vi "Calculate_Global_Cost_F()-3.vi"(6 "[IN] Max angle":dbl, 7 "[IN] Subtracks in Row":T1(array[cluster]), 8 "error IN":errorcluster, 9 "[IN] Areas particles\nPrimary Detected":dbl[][](array[numeric]), 10 "[IN] Primary \n(X,Y) Detected":dbl[][](array[numeric]), 11 "[IN] Cost function":i8[](array[numeric])) -> (0 "error OUT":errorcluster, 3 "[OUT] Cost function":i8[](array[numeric]))   [LabVIEW 2013]
uses:
  <vilib>/Analysis/NI_AALBase.lvlib
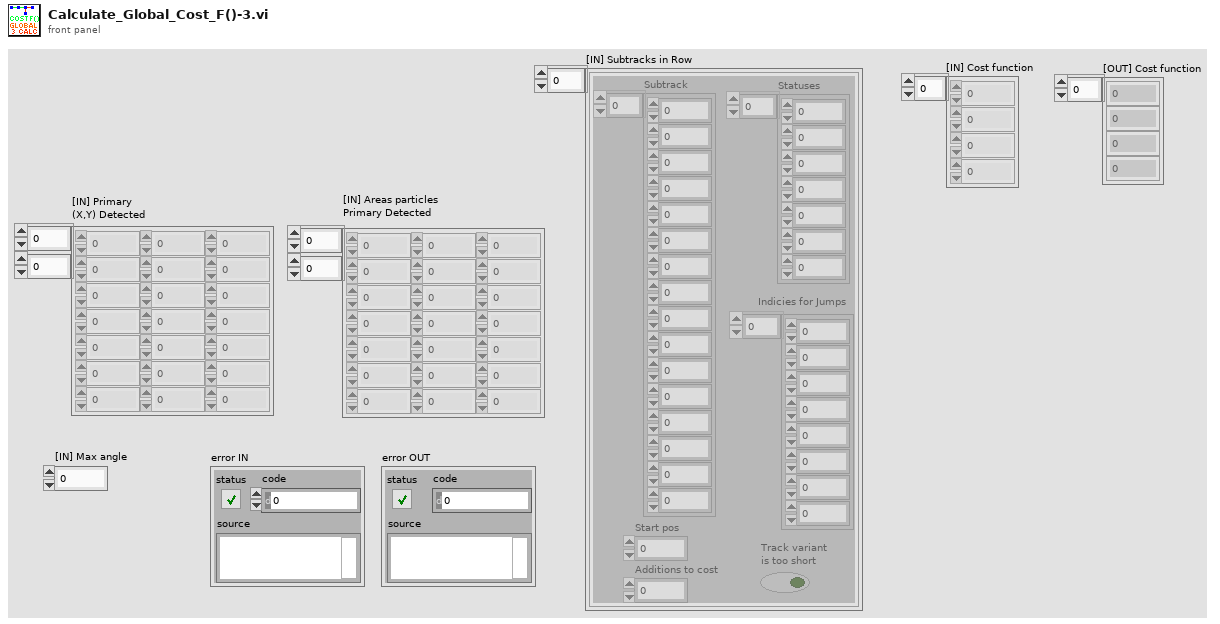
[diagram p1: front panel]
types:
  T1 = cluster{"Subtrack":dbl[], "Statuses":i16[], "Start pos":i32, "Additions to cost":i8, "Track variant \nis too short":bool, "Indicies for Jumps":i32[]}[]
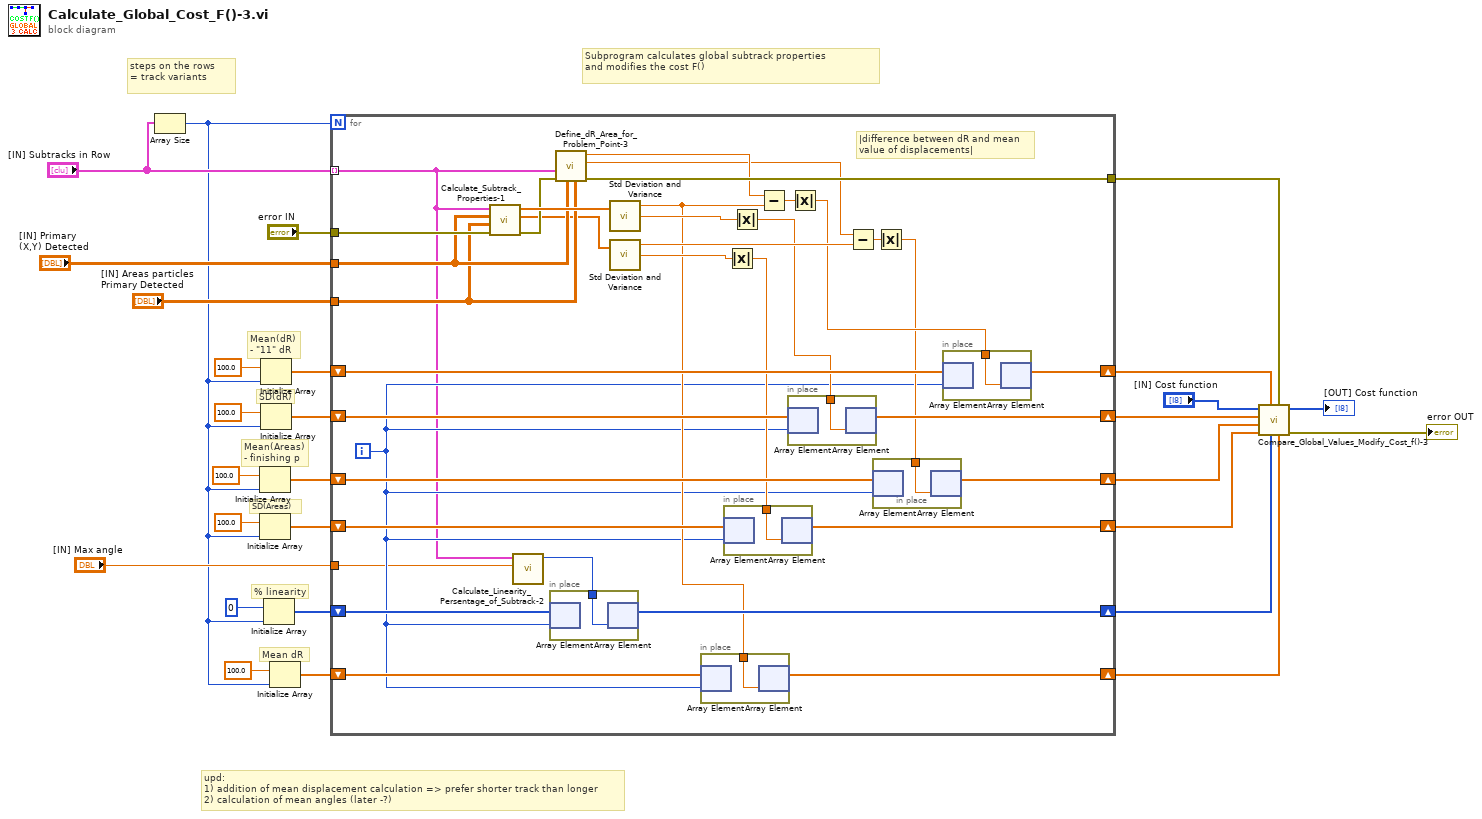
[diagram p0: block diagram]
diagram:
  # "upd: \n1) addition of mean displacement calculation => prefer shorter track than longer \n2) calculation of mean angles (later -?)"
  # "Mean dR"
  # "Subprogram calculates global subtrack properties\nand modifies the cost F()"
  # "Mean(Areas)\n- finishing p"
  # "SD(Areas)"
  # "% linearity"
  # "Mean(dR)\n- \"11\" dR"
  # "SD(dR)"
  # "steps on the rows\n= track variants"
  n1 = Array Size(array="[IN] Subtracks in Row") -> (size(s)=w3:i32)
  n2 = Initialize Array(100.0, w3) -> (w18:dbl[])
  n3 = Initialize Array(100.0, w3) -> (w17:dbl[])
  n4 = Initialize Array(100.0, w3) -> (w26:dbl[])
  n5 = Initialize Array(100.0, w3) -> (w25:dbl[])
  n6 = Initialize Array(u8 0, w3) -> (w15:u8[])
  n7 = Initialize Array(100.0, w3) -> (w2:dbl[])
  n8 = for {
    N: w3 -> [_]
    shift-right: [w48] -> w12
    shift-left: w26 -> [w49]
    shift-right: [w45] -> w5
    shift-left: w25 -> [w47]
    tunnel: "error IN" -> [w63]
    tunnel: "[IN] Primary \n(X,Y) Detected" -> [w53]
    tunnel: "[IN] Areas particles\nPrimary Detected" -> [w52]
    shift-right: [w42] -> w6
    shift-left: w18 -> [w44]
    shift-right: [w39] -> w7
    shift-left: w17 -> [w41]
    tunnel: "[IN] Max angle" -> [w30]
    shift-right: [w37] -> w8
    shift-left: w15 -> [w38]
    tunnel: [w55] -> w11
    tunnel: "[IN] Subtracks in Row" -> [w31] mode=indexing
    shift-right: [w33] -> w1
    shift-left: w2 -> [w35]
    i -> [w32]
    # "|difference between dR and mean\nvalue of displacements|"
    n9 = call "Calculate_Subtrack_Properties-1.vi"("error IN"=w63, "[IN] Areas particles\nPrimary Detected"=w52, "[IN] Primary \n(X,Y) Detected"=w53, "[IN] Subtrack"=w31) -> ("error OUT"=w56:errorcluster, "[OUT] Areas"=w36:dbl[], "[OUT] dR (displ)"=w62:dbl[])  [unwired: 2 in, 1 out]
    n10 = call "Calculate_Linearity_Persentage_of_Subtrack-2.vi"("[IN] Max angle"=w30, "[IN] Subtrack"=w31) -> ("[OUT] Track Linearity in %"=w29:u8)  [unwired: 5 in]
    n11 = in-place {
      in-place-border: w29 -> [w65]
      n12 = in-place-array #1(w38, w32) -> ()  [unwired: 1 out]
      n13 = in-place-array #1(w65) -> (w37:u8[])  [unwired: 1 out]
    }
    n14 = call "Define_dR_Area_for_Problem_Point-3.vi"("[IN] Areas particles\nPrimary Detected"=w52, "[IN] Primary \n(X,Y) Detected"=w53, "error IN"=w56, "[IN] Subtrack"=w31) -> ("error OUT"=w55:errorcluster, "[OUT] Area Problem Point\n101 - Starting Point\n11 - Ending Point"=w51:dbl, "[OUT] dR for Problem Point"=w54:dbl)  [unwired: 5 in]
    n15 = call <vilib>:"Std Deviation and Variance.vi"("X"=w62) -> ("mean"=w34:dbl, "standard deviation"=w61:dbl)  [unwired: 1 in, 1 out]
    n16 = call <vilib>:"Std Deviation and Variance.vi"("X"=w36) -> ("mean"=w58:dbl, "standard deviation"=w60:dbl)  [unwired: 1 in, 1 out]
    n17 = in-place {
      in-place-border: w34 -> [w64]
      n18 = in-place-array #2(w35, w32) -> ()  [unwired: 1 out]
      n19 = in-place-array #2(w64) -> (w33:dbl[])  [unwired: 1 out]
    }
    n20 = Absolute Value(x=w60) -> (abs(x)=w40:dbl)
    n21 = in-place {
      in-place-border: w40 -> [w66]
      n22 = in-place-array #3(w41, w32) -> ()  [unwired: 1 out]
      n23 = in-place-array #3(w66) -> (w39:dbl[])  [unwired: 1 out]
    }
    n24 = Absolute Value(x=w61) -> (abs(x)=w46:dbl)
    n25 = Subtract(x=w54, y=w34) -> (x-y=w59:dbl)
    n26 = in-place {
      in-place-border: w46 -> [w68]
      n27 = in-place-array #4(w47, w32) -> ()  [unwired: 1 out]
      n28 = in-place-array #4(w68) -> (w45:dbl[])  [unwired: 1 out]
    }
    n29 = Absolute Value(x=w59) -> (abs(x)=w50:dbl)
    n30 = Subtract(x=w51, y=w58) -> (x-y=w57:dbl)
    n31 = Absolute Value(x=w57) -> (abs(x)=w43:dbl)
    n32 = in-place {
      in-place-border: w43 -> [w67]
      n33 = in-place-array #5(w44, w32) -> ()  [unwired: 1 out]
      n34 = in-place-array #5(w67) -> (w42:dbl[])  [unwired: 1 out]
    }
    n35 = in-place {
      in-place-border: w50 -> [w69]
      n36 = in-place-array #6(w49, w32) -> ()  [unwired: 1 out]
      n37 = in-place-array #6(w69) -> (w48:dbl[])  [unwired: 1 out]
    }
  }
  n38 = call "Compare_Global_Values_Modify_Cost_f()-3.vi"("[IN] Mean dR"=w1, "error IN"=w11, "[IN] Linearity"=w8, "[IN] Array of Mean\n(dR) - Problem dR"=w12, "[IN] SD(Areas)"=w7, "[IN] Array of Mean(Areas)\n - Problem finish Area"=w6, "[IN] SD(dR)"=w5, "[IN] Cost function"="[IN] Cost function") -> ("error OUT"=→"error OUT":errorcluster, "[OUT] Cost function"=→"[OUT] Cost function":i8[])  [unwired: 2 in]
